vi "VoltageRatioInput Voltage Ratio Event Example.vi"() -> ()   [LabVIEW 2012, in "Phidget Voltage Ratio Input.lvlib"]
uses:
  <instrlib>/Phidgets/Phidget Voltage Ratio Input/Phidget Voltage Ratio Input.lvlib
  <instrlib>/Phidgets/Phidget Voltage Ratio Input/Public/VoltageRatioInputStart.vi
  <instrlib>/Phidgets/Phidget Voltage Ratio Input/Public/VoltageRatioInputClose.vi
  <instrlib>/Phidgets/Phidget Common/Phidget Common.lvlib
panel:
  in  "IsHubPort":bool
  out "Voltage Ratio":dbl format="%_4g"
  in  "stop":bool
  out "Serial Number Return":i32
  in  "Device Info":T1={"Serial Number"=-1, "Channel"=0, "Port"=0}
  out "error out":errorcluster
  # "Be sure to use this stop button to stop the program.\nIf you use the \"Abort Execution\" button, you will\nneed to use PhidgetResetLibrary.vi or restart Labview \nin order for any Phidgets to work."
  # "Yes\n\nNo"
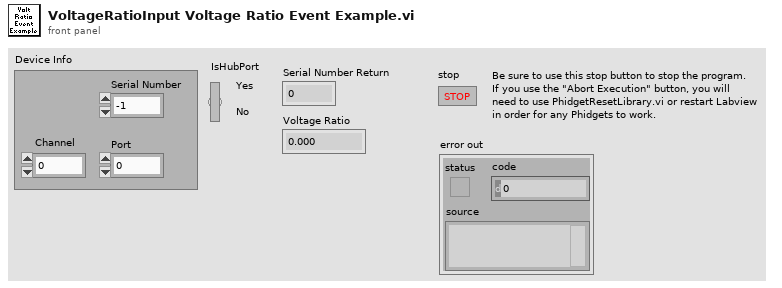
[diagram p1: front panel]
types:
  T1 = cluster{"Serial Number":i32, "Channel":i32, "Port":i32}
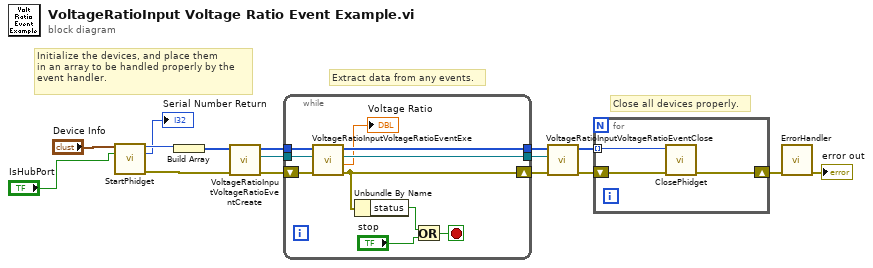
[diagram p0: block diagram]
diagram:
  # "Close all devices properly."
  # "Extract data from any events."
  # "Initialize the devices, and place them\nin an array to be handled properly by the\nevent handler."
  n1 = call-poly <instrlib>:"StartPhidget.vi"("Device Info"="Device Info", "IsHubPort"="IsHubPort") -> ("Phidget ID"=w6:u64, "Serial Number Return"=→"Serial Number Return":i32, "error out"=w2:errorcluster)  [unwired: 10 in, 1 out]
  n2 = Build Array(w6) -> (w16:u64[])
  n3 = call <instrlib>:"VoltageRatioInputVoltageRatioEventCreate.vi"("error in (no error)"=w2, "Devices In"=w16) -> ("error out"=w9:errorcluster, "Event Registration Refnum"=w14:refnum<event-registration>, "Devices Out"=w15:u64[])  [unwired: 7 in]
  n4 = while {
    tunnel: w15 -> [w26]
    tunnel: w14 -> [w22]
    tunnel: [w25] -> w11
    shift-right: [w21] -> w10
    shift-left: w9 -> [w24]
    tunnel: [w23] -> w4
    stop <- w20 stop-if-true
    n5 = call <instrlib>:"VoltageRatioInputVoltageRatioEventExe.vi"("error in (no error)"=w24, "Event Registration Refnum In"=w22, "Devices In"=w26) -> ("error out"=w21:errorcluster, "VoltageRatio"=→"Voltage Ratio":dbl, "Event Registration Refnum Out"=w25:refnum<event-registration>, "Devices Out"=w23:u64[])  [unwired: 2 in, 3 out]
    n6 = Unbundle By Name(w21) -> ("status"=w18:bool)
    n7 = Or(x=w18, y="stop") -> (x .or. y?=w20:bool)
  }
  n8 = call <instrlib>:"VoltageRatioInputVoltageRatioEventClose.vi"("error in (no error)"=w10, "Event Registration Refnum In"=w11, "Devices In"=w4) -> ("error out"=w7:errorcluster, "Devices Out"=w5:u64[])  [unwired: 7 in]
  n9 = for {
    tunnel: w5 -> [w27] mode=indexing
    shift-right: [w29] -> w13
    shift-left: w7 -> [w28]
    n10 = call-poly <instrlib>:"ClosePhidget.vi"("error in"=w28, "Device In"=w27) -> ("error out"=w29:errorcluster)  [unwired: 9 in]
  }
  n11 = call <instrlib>:"ErrorHandler.vi"("error in"=w13) -> ("error out"=→"error out":errorcluster)  [unwired: 9 in, 1 out]
